vi "Determine Next Generation Level.vi"(8 "error in (no error)":errorcluster, 10 "current generation level":dbl, 11 "measurement configuration":T1 {"acq sampling rate" format="%0.2f"; "master clock rate" format="%#_6pHz"; "frame clock rate" format="%#_6pHz"}) -> (0 "error out":errorcluster, 3 "next generation level":dbl)   [LabVIEW 2021, in "Stepped Frequency Sweep_Class D Amplifier.lvlib"]
uses:
  Stepped Frequency Sweep_Class D Amplifier.lvlib
  Measurement Configuration.ctl
  shared/controls/digital audio protocol/data justification.ctl
  shared/controls/digital audio protocol/endianness.ctl
  shared/controls/digital audio protocol/digital edge.ctl
  shared/controls/digital audio protocol/logic level.ctl
  shared/controls/digital output level units.ctl
  shared/controls/weighting filter.ctl
  shared/controls/highpass filter.ctl
  shared/controls/lowpass filter.ctl
  shared/controls/sweep profile.ctl
  shared/controls/units - snr.ctl
  shared/controls/units - ratio.ctl
  shared/controls/regulation target.ctl
  shared/controls/regulation target value units.ctl
  shared/controls/audio controls.lvlib
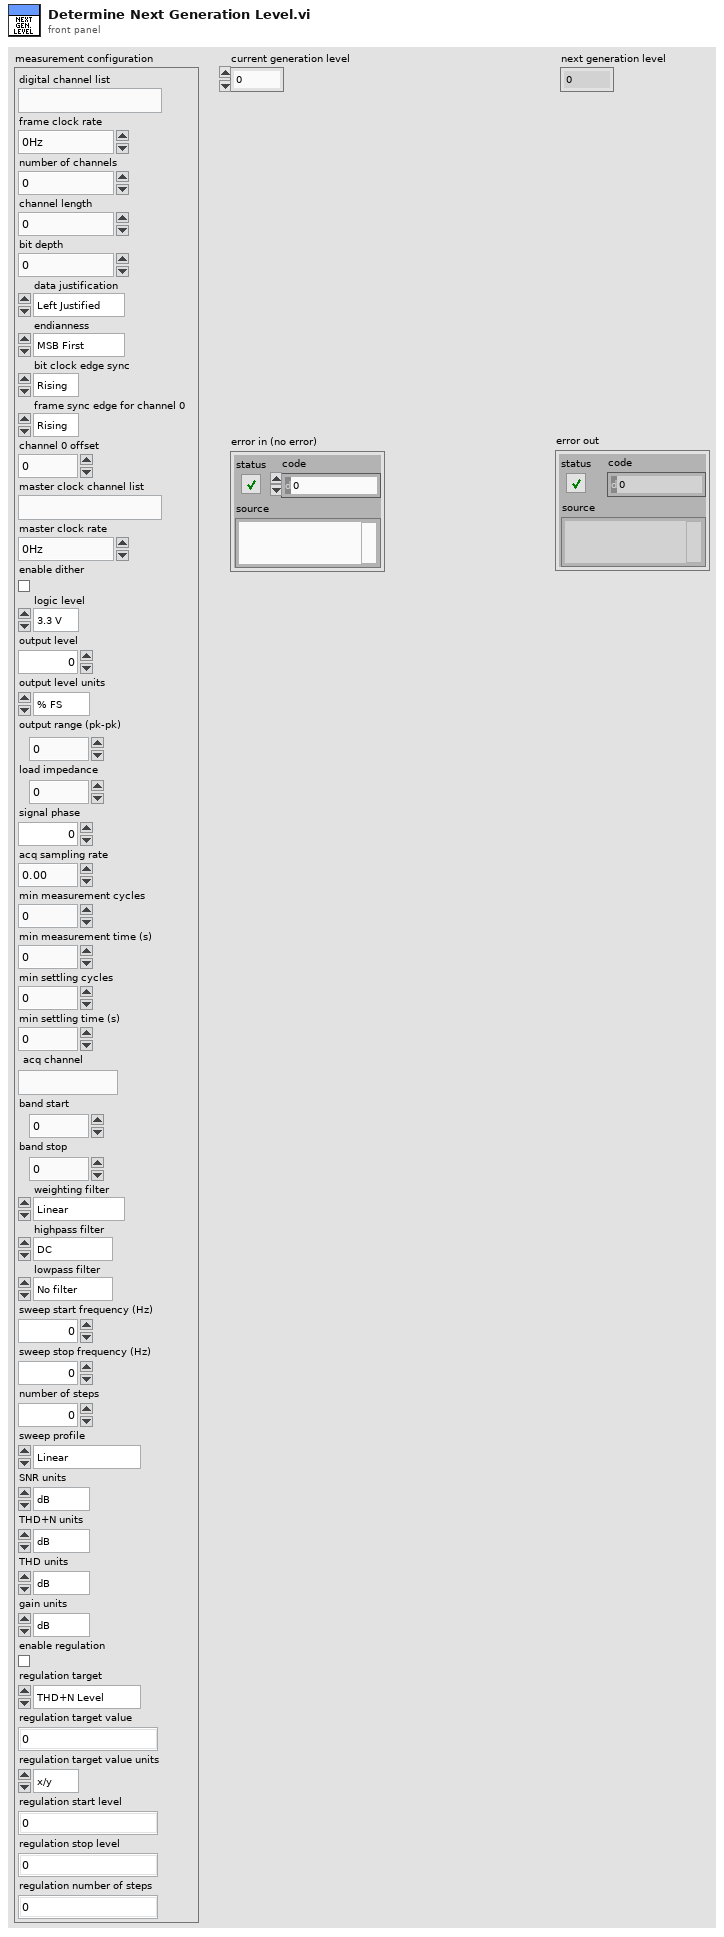
[diagram p1: front panel]
types:
  T1 = typedef "Stepped Frequency Sweep_Class D Amplifier.lvlib/Measurement Configuration.ctl" = cluster{"digital channel list":string, "frame clock rate":dbl, "number of channels":u32, "channel length":u32, "bit depth":u32, "data justification":T2, "endianness":T3, "bit clock edge sync":T4, "frame sync edge for channel 0":T4, "channel 0 offset":u32, "master clock channel list":string, "master clock rate":dbl, "enable dither":bool, "logic level":T5, "output level":dbl, "output level units":T6, "output range (pk-pk)":dbl, "load impedance":dbl, "signal phase":dbl, "acq sampling rate":dbl, "min measurement cycles":u32, "min measurement time (s)":dbl, "min settling cycles":u32, "min settling time (s)":dbl, "acq channel":string, "band start":dbl, "band stop":dbl, "weighting filter":T7, "highpass filter":T8, "lowpass filter":T9, "sweep start frequency (Hz)":dbl, "sweep stop frequency (Hz)":dbl, "number of steps":u32, "sweep profile":T10, "SNR units":T11, "THD+N units":T12, "THD units":T12, "gain units":T12, "enable regulation":bool, "regulation target":T13, "regulation target value":dbl, "regulation target value units":T14, "regulation start level":dbl, "regulation stop level":dbl, "regulation number of steps":u32}
  T2 = typedef "data justification.ctl" = enum32{"Left Justified", "Right Justified"}
  T3 = typedef "endianness.ctl" = enum32{"MSB First", "LSB First"}
  T4 = typedef "digital edge.ctl" = enum32{"Rising", "Falling"}
  T5 = typedef "logic level.ctl" = enum32{"3.3 V", "1.8 V", "1.2 V"}
  T6 = typedef "audio controls.lvlib/digital output level units.ctl" = enum32{"% FS", "dBFS"}
  T7 = typedef "weighting filter.ctl" = enum32{"Linear", "A-weighting", "B-weighting", "C-weighting"}
  T8 = typedef "highpass filter.ctl" = enum32{"DC", "AC"}
  T9 = typedef "lowpass filter.ctl" = enum32{"No filter", "AES17 20kHz", "AES17 40kHz"}
  T10 = typedef "audio controls.lvlib/sweep profile.ctl" = enum32{"Linear", "Logarithmic"}
  T11 = typedef "audio controls.lvlib/units - snr.ctl" = enum32{"dB", "x/y"}
  T12 = typedef "audio controls.lvlib/units - ratio.ctl" = enum32{"dB", "%", "x/y"}
  T13 = typedef "regulation target.ctl" = enum32{"THD+N Level", "THD+N Ratio", "RMS Level", "RMS Ratio", "Output Power"}
  T14 = typedef "regulation target value units.ctl" = enum32{"x/y", "%", "dB", "Vrms", "W"}
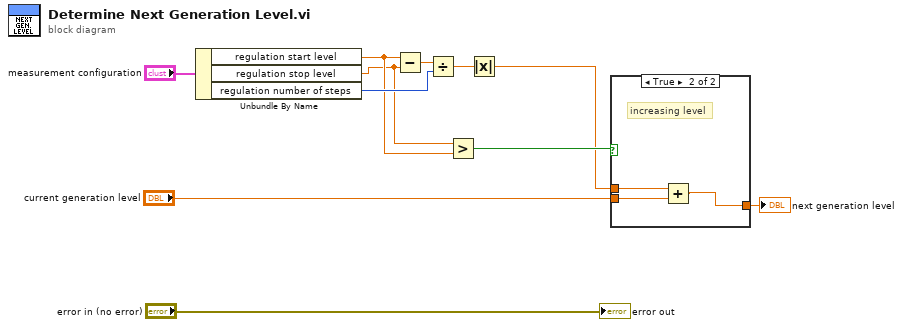
[diagram p0: block diagram]
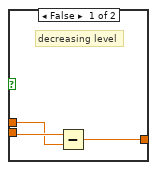
[diagram p2: hidden frame]
diagram:
  n1 = Unbundle By Name("measurement configuration") -> ("regulation start level"=w5:dbl, "regulation stop level"=w4:dbl, "regulation number of steps"=w8:u32)
  n2 = Subtract(x=w5, y=w4) -> (x-y=w9:dbl)
  n3 = Divide(x=w9, y=w8) -> (x/y=w6:dbl)
  n4 = Greater?(x=w4, y=w5) -> (0:w3:bool)
  n5 = Absolute Value(x=w6) -> (abs(x)=w1:dbl)
  n6 = case shown="True" w3 {
    tunnel: "current generation level" -> [w14 w17]
    tunnel: w1 -> [w13 w16]
    tunnel: [w12 w15] -> w2
    frame False {
      # "decreasing level"
      n7 = Subtract(x=w14, y=w13) -> (x-y=w12:dbl)
    }
    frame True {
      # "increasing level"
      n8 = Add(x=w16, y=w17) -> (x+y=w15:dbl)
    }
  }
  "next generation level" <- w2
  "error out" <- "error in (no error)"
